vi "Read RFFE Address.vi"(8 "error in (no error)":errorcluster, 11 "Toggle 6 in":refnum<class "Toggle 6.lvclass">) -> (0 "error out":errorcluster, 2 "RFFE Adress":u32=7 min=6 max=7 step=1, 3 "Toggle 6 out":refnum<class "Toggle 6.lvclass">)   [LabVIEW 2020, in "Toggle 6.lvclass"]
uses:
  Toggle 6.lvclass
  Toggle 6.lvclass/Toggle 6.ctl
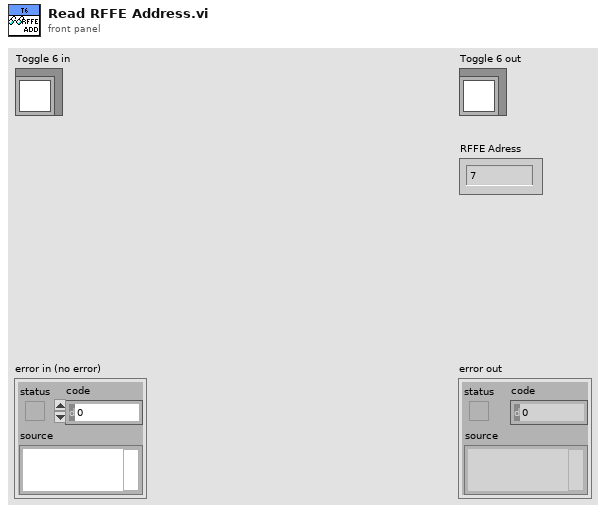
[diagram p1: front panel]
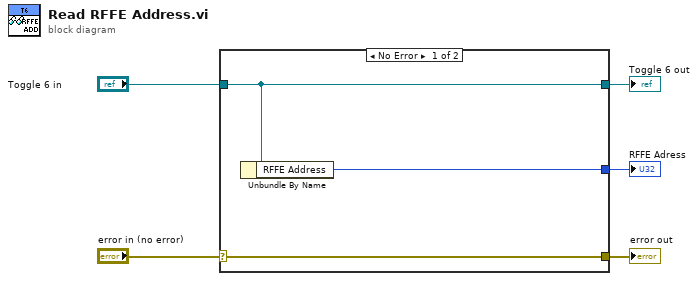
[diagram p0: block diagram]
diagram:
  n1 = case shown="No Error" "error in (no error)" {
    selector: "error in (no error)" -> [w8 w9]
    tunnel: [w8 w9] -> w4
    tunnel: [w7 w10] -> w2
    tunnel: "Toggle 6 in" -> [w7 w10]
    tunnel: [w6 _] -> w1
    frame No Error {
      n2 = Unbundle By Name(w7) -> ("RFFE Address"=w6:u32)
    }
    frame Error {
    }
  }
  "error out" <- w4
  "Toggle 6 out" <- w2
  "RFFE Adress" <- w1
